vi "Kinesis-program.vi"() -> ()   [LabVIEW 2014]
doc: "André Romero - 2017\nandretec@ifsc.usp.br"
panel:
  out "Numeric 2":i32
  out "GetPOS":dbl format="%#_6e"
  out "Numeric":i32
  out "IsMoving":bool
  out "GetPOS Y":dbl=10.0
  out "GetPOS X":dbl=10.0 format="%^#1_6e"
  in  "GO Move":bool
  out "Motor 2":bool
  out "Motor 1":bool
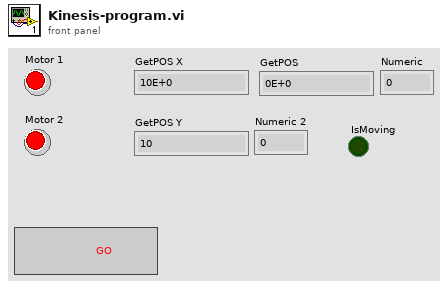
[diagram p1: front panel]
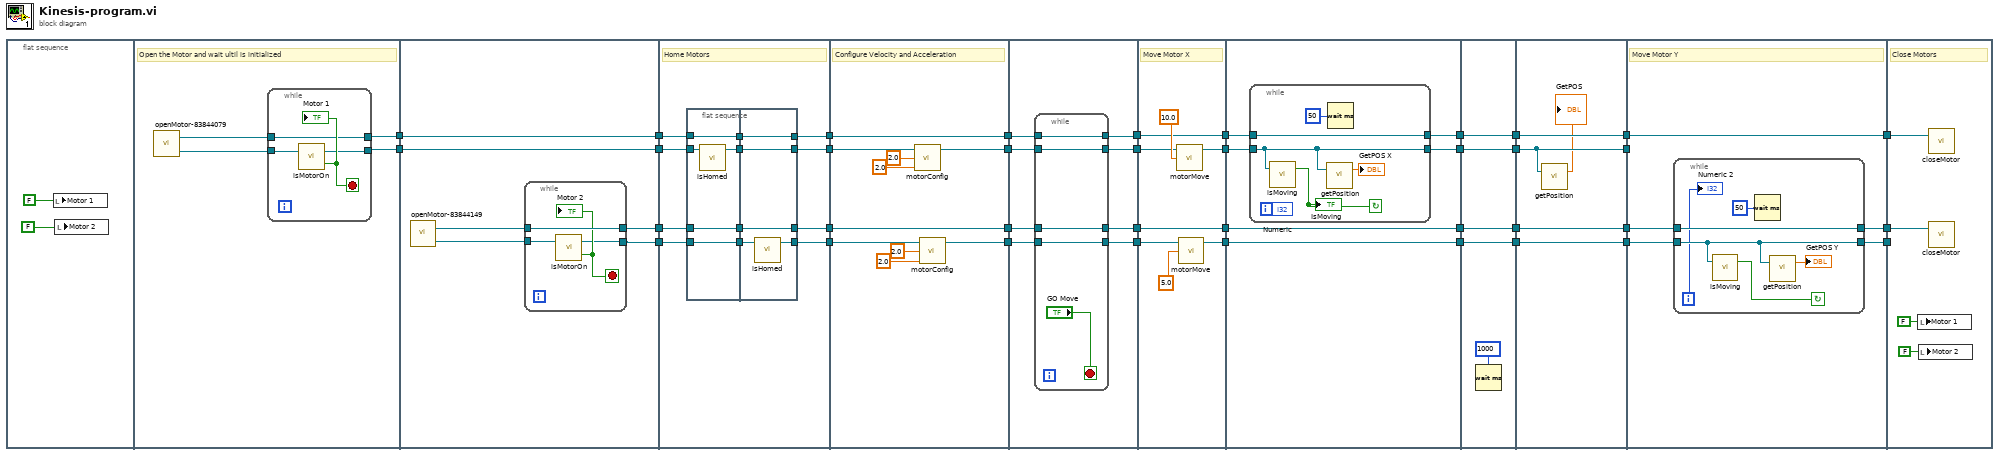
[diagram p0: block diagram]
diagram:
  n1 = flat-sequence {
    tunnel: [w43] -> w6
    tunnel: [w42] -> w4
    tunnel: w6 -> [w53]
    tunnel: [w53] -> w5
    tunnel: w4 -> [w52]
    tunnel: [w52] -> w3
    tunnel: [w51] -> w2
    tunnel: [w50] -> w1
    tunnel: w5 -> [w65]
    tunnel: w3 -> [w64]
    tunnel: [w67] -> w35
    tunnel: w2 -> [w66]
    tunnel: [w68] -> w33
    tunnel: w1 -> [w69]
    tunnel: [w61] -> w37
    tunnel: [w60] -> w31
    tunnel: w37 -> [w88]
    tunnel: [w88] -> w36
    tunnel: w35 -> [w89]
    tunnel: [w89] -> w34
    tunnel: w33 -> [w87]
    tunnel: [w84] -> w32
    tunnel: w31 -> [w80]
    tunnel: [w81] -> w30
    tunnel: w36 -> [w97]
    tunnel: [w96] -> w23
    tunnel: w34 -> [w93]
    tunnel: [w90] -> w26
    tunnel: w32 -> [w91]
    tunnel: [w92] -> w25
    tunnel: w30 -> [w94]
    tunnel: [w95] -> w24
    tunnel: w26 -> [w110]
    tunnel: [w110] -> w22
    tunnel: w25 -> [w105]
    tunnel: [w104] -> w21
    tunnel: w24 -> [w107]
    tunnel: [w106] -> w20
    tunnel: w23 -> [w108]
    tunnel: [w108] -> w19
    tunnel: w22 -> [w112]
    tunnel: [w112] -> w18
    tunnel: w21 -> [w111]
    tunnel: w20 -> [w113]
    tunnel: [w114] -> w17
    tunnel: w19 -> [w116]
    tunnel: [w115] -> w16
    tunnel: [w111] -> w7
    tunnel: w18 -> [w127]
    tunnel: [w127] -> w15
    tunnel: [w126] -> w13
    tunnel: w17 -> [w125]
    tunnel: [w125] -> w11
    tunnel: w16 -> [w124]
    tunnel: [w124] -> w9
    tunnel: w7 -> [w126]
    tunnel: w15 -> [w132]
    tunnel: [w132] -> w14
    tunnel: w13 -> [w131]
    tunnel: [w131] -> w12
    tunnel: w11 -> [w129]
    tunnel: [w129] -> w10
    tunnel: w9 -> [w130]
    tunnel: [w130] -> w8
    tunnel: w14 -> [w137]
    tunnel: [w136] -> w29
    tunnel: w12 -> [w133]
    tunnel: [w135] -> w28
    tunnel: w10 -> [_]
    tunnel: w8 -> [w134]
    tunnel: [w134] -> w27
    tunnel: w29 -> [w146]
    tunnel: w28 -> [_]
    tunnel: w27 -> [w147]
    frame #0 {
      n2 = local write "Motor 1"(FALSE ("isConnected")) -> ()
      n3 = local write "Motor 2"(FALSE ("isConnected 2")) -> ()
    }
    frame #1 {
      # "Open the Motor and wait ultil is initialized"
      n4 = call "openMotor-83844079.vi"() -> ("Device"=w41:refnum<k24>, ".NET Refnum out"=w40:refnum<k24>)  [unwired: 2 in]
      n5 = while {
        tunnel: [w46] -> w43
        tunnel: [w44] -> w42
        tunnel: w40 -> [w46]
        tunnel: w41 -> [w45]
        stop <- w47 stop-if-true
        n6 = call "isMotorOn.vi"("Device"=w45) -> ("isConnected"=w47:bool, "Device out"=w44:refnum<k24>)  [unwired: 1 in]
        "Motor 1" <- w47
      }
    }
    frame #2 {
      n7 = call "openMotor-83844149.vi"() -> ("Device"=w48:refnum<k24>, ".NET Refnum out"=w49:refnum<k24>)  [unwired: 2 in]
      n8 = while {
        tunnel: w48 -> [w55]
        tunnel: [w57] -> w51
        tunnel: w49 -> [w57]
        tunnel: [w54] -> w50
        stop <- w56 stop-if-true
        n9 = call "isMotorOn.vi"("Device"=w55) -> ("isConnected"=w56:bool, "Device out"=w54:refnum<k24>)  [unwired: 1 in]
        "Motor 2" <- w56
      }
    }
    frame #3 {
      # "Home Motors"
      n10 = flat-sequence {
        tunnel: w69 -> [w70]
        tunnel: w66 -> [w74]
        tunnel: w65 -> [w73]
        tunnel: w64 -> [w72]
        tunnel: [w74] -> w63
        tunnel: [w73] -> w62
        tunnel: [w71] -> w59
        tunnel: [w70] -> w58
        tunnel: [w77] -> w60
        tunnel: [w78] -> w61
        tunnel: [w79] -> w67
        tunnel: [w75] -> w68
        tunnel: w63 -> [w79]
        tunnel: w62 -> [w78]
        tunnel: w59 -> [w77]
        tunnel: w58 -> [w76]
        frame #0 {
          n11 = call "isHomed.vi"("Device in"=w72) -> ("Device out"=w71:refnum<k24>)  [unwired: 4 in]
        }
        frame #1 {
          n12 = call "isHomed.vi"("Device in"=w76) -> ("Device out"=w75:refnum<k24>)  [unwired: 4 in]
        }
      }
    }
    frame #4 {
      # "Configure Velocity and Acceleration"
      n13 = call "motorConfig.vi"("Velocity"=2.0 ("MaxVelocity"), "Acceleration"=2.0, "Device in"=w80) -> ("Device out"=w81:refnum<k24>)  [unwired: 2 in]
      n14 = call "motorConfig.vi"("Velocity"=2.0 ("MaxVelocity"), "Acceleration"=2.0, "Device in"=w87) -> ("Device out"=w84:refnum<k24>)  [unwired: 2 in]
    }
    frame #5 {
      n15 = while {
        tunnel: [w101] -> w96
        tunnel: w97 -> [w101]
        tunnel: [w100] -> w95
        tunnel: w94 -> [w100]
        tunnel: w93 -> [w98]
        tunnel: [w99] -> w92
        tunnel: w91 -> [w99]
        tunnel: [w98] -> w90
        stop <- "GO Move" stop-if-true
      }
    }
    frame #6 {
      # "Move Motor X"
      n16 = call "motorMove.vi"("position"=10.0, "Device in"=w107) -> ("Device out"=w106:refnum<k24>)  [unwired: 3 in]
      n17 = call "motorMove.vi"("position"=5.0, "Device in"=w105) -> ("Device out"=w104:refnum<k24>)  [unwired: 3 in]
    }
    frame #7 {
      n18 = while {
        tunnel: w116 -> [w122]
        tunnel: w113 -> [w121]
        tunnel: [w122] -> w115
        tunnel: [w121] -> w114
        i -> [w118]
        stop <- w120 continue-if-true
        n19 = call "isMoving.vi"("Device in"=w121) -> ("IsMoving"=w120:bool)  [unwired: 2 in]
        "IsMoving" <- w120
        n20 = call "getPosition.vi"("Device"=w121) -> ("GetPOS"=→"GetPOS X":dbl)  [unwired: 2 in]
        n21 = Wait (ms)(milliseconds to wait=u32 50) -> ()  [unwired: 1 out]
        "Numeric" <- w118
      }
    }
    frame #8 {
      n22 = Wait (ms)(milliseconds to wait=u32 1000) -> ()  [unwired: 1 out]
    }
    frame #9 {
      n23 = call "getPosition.vi"("Device"=w129) -> ("GetPOS"=→"GetPOS":dbl)  [unwired: 2 in]
    }
    frame #10 {
      # "Move Motor Y"
      n24 = while {
        tunnel: w137 -> [w143]
        tunnel: w133 -> [w142]
        tunnel: [w143] -> w136
        tunnel: [w142] -> w135
        i -> [w138]
        stop <- w141 continue-if-true
        n25 = call "isMoving.vi"("Device in"=w142) -> ("IsMoving"=w141:bool)  [unwired: 2 in]
        n26 = Wait (ms)(milliseconds to wait=u32 50) -> ()  [unwired: 1 out]
        n27 = call "getPosition.vi"("Device"=w142) -> ("GetPOS"=→"GetPOS Y":dbl)  [unwired: 2 in]
        "Numeric 2" <- w138
      }
    }
    frame #11 {
      # "Close Motors"
      n28 = local write "Motor 1"(FALSE ("Motor 1")) -> ()
      n29 = local write "Motor 2"(FALSE ("Motor 2")) -> ()
      n30 = call "closeMotor.vi"(".NET Refnum in"=w147) -> ()  [unwired: 2 in]
      n31 = call "closeMotor.vi"(".NET Refnum in"=w146) -> ()  [unwired: 2 in]
    }
  }
